vi "SetFrameBounds.vi"(8 "error in (no error)":errorcluster, 11 "menu in":refnum<class "menu.lvclass">) -> (0 "error out":errorcluster, 3 "menu out":refnum<class "menu.lvclass">)   [LabVIEW 2009, in "menu.lvclass"]
uses:
  menu.lvclass
  menu.lvclass/menu.ctl
  Frame/frame.lvclass
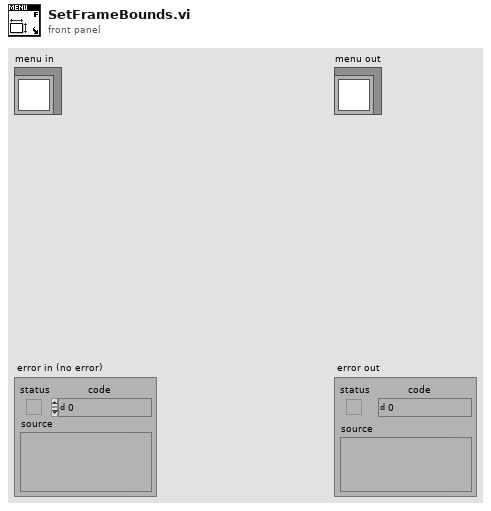
[diagram p1: front panel]
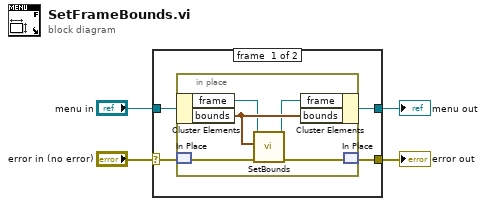
[diagram p0: block diagram]
diagram:
  n1 = case shown="No Error" "error in (no error)" {
    selector: "error in (no error)" -> [w7 w15]
    tunnel: [w6 w15] -> w1
    tunnel: [w5 w14] -> w3
    tunnel: "menu in" -> [w8 w14]
    frame #0 {
      n2 = in-place {
        n3 = in-place-cluster #1(w8) -> ("frame"=w12:refnum<class "frame.lvclass">, "bounds"=w13:cluster{"width":u32, "height":u32})
        n4 = in-place-match #2(w7) -> (w9:errorcluster)
        n5 = call "SetBounds.vi"("error in (no error)"=w9, "bounds"=w13, "frame in"=w12) -> ("error out"=w10:errorcluster, "frame out"=w11:refnum<class "frame.lvclass">)  [unwired: 7 in]
        n6 = in-place-cluster #1("frame"=w11, "bounds"=w13) -> (w5:refnum<class "menu.lvclass">)
        n7 = in-place-match #2(w10) -> (w6:errorcluster)
      }
    }
    frame #1 {
    }
  }
  "menu out" <- w3
  "error out" <- w1
